vi "TestModel.vi"() -> ()   [LabVIEW 2015]
uses:
  CustomControl/Model.ctl
panel:
  in  "OK Button":bool
  in  "TestModel":T1
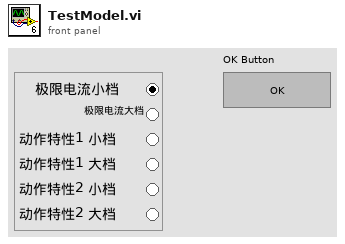
[diagram p1: front panel]
types:
  T1 = typedef "Model.ctl" = enum32{"lowLimit", "upLimit", "lowAction1", "upAction1", "lowAction2", "upAction2"}
  T2 = enum8{"Enabled", "Disabled", "Disabled and Grayed Out"}
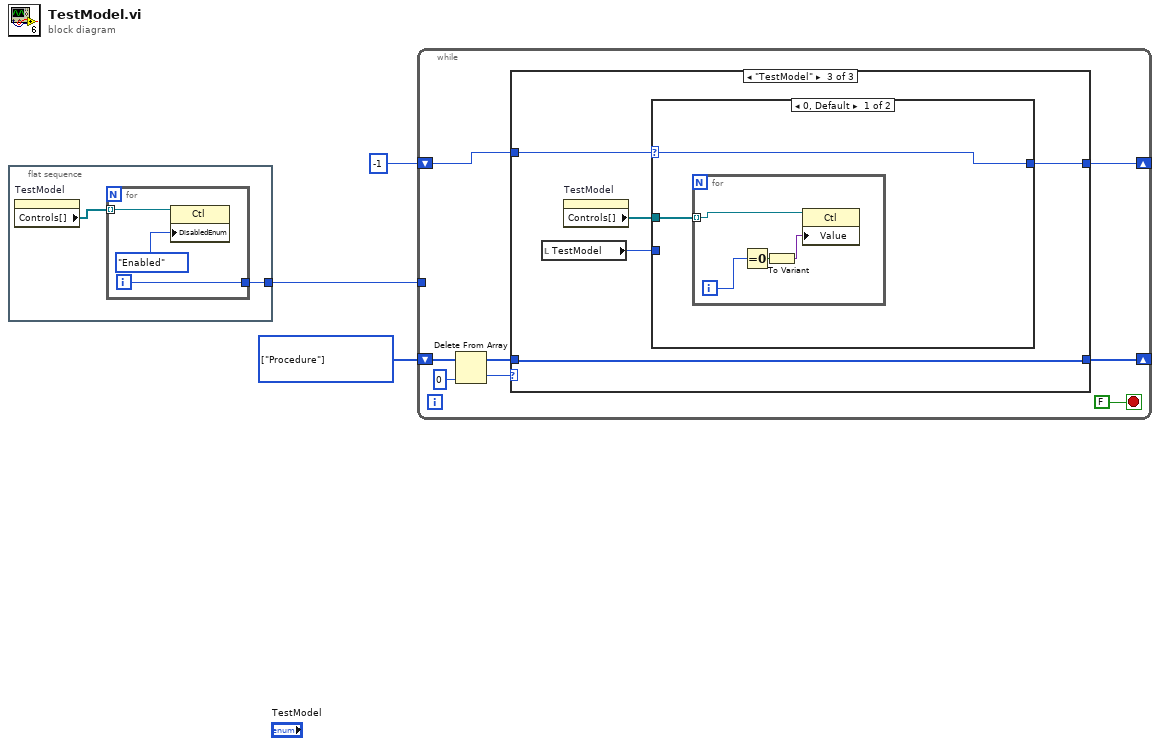
[diagram p0: block diagram]
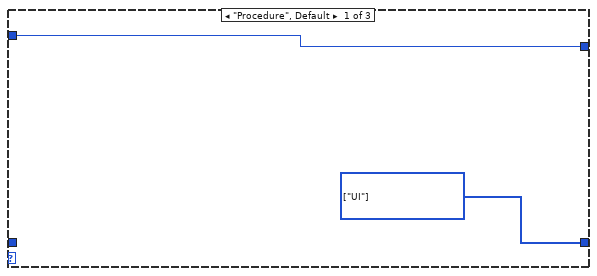
[diagram p2: hidden frame]
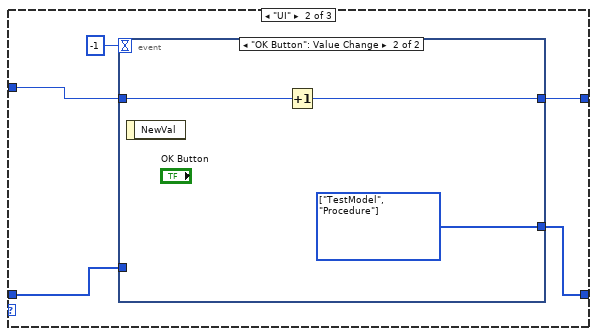
[diagram p3: hidden frame]
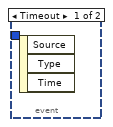
[diagram p4: hidden frame]
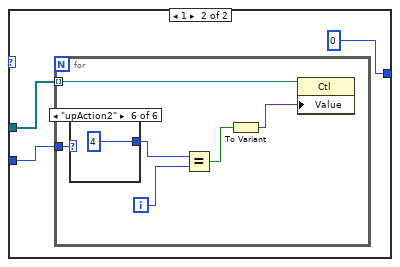
[diagram p5: hidden frame]
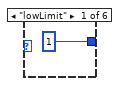
[diagram p6: hidden frame]
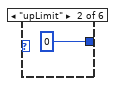
[diagram p7: hidden frame]
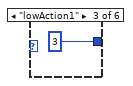
[diagram p8: hidden frame]
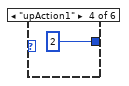
[diagram p9: hidden frame]
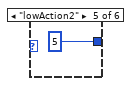
[diagram p10: hidden frame]
diagram:
  w2 = enum16{"Procedure", "UI", "TestModel"}[] [enum."Procedure"] items=["Procedure", "UI", "TestModel"]
  n1 = flat-sequence {
    tunnel: [w4] -> w1
    frame #0 {
      n2 = property on="TestModel" class="RadioBtnsControl (strict)"() -> ("Controls[]"=w5:refnum<vi>[])  [unwired: 2 in, 2 out]
      n3 = for {
        tunnel: w5 -> [w8] mode=indexing
        tunnel: [w6] -> w4
        i -> [w6]
        n4 = property class="Ctl"(reference=w8, "DisabledEnum"=T2."Enabled" ("Disabled")) -> ()  [unwired: 1 in, 2 out]
      }
    }
  }
  n5 = while {
    shift-right: [w14] -> _
    shift-left: -1 -> [w15]
    shift-right: [w10] -> _
    shift-left: w2 -> [w13]
    tunnel: w1 -> [_]
    stop <- FALSE stop-if-true
    n6 = Delete From Array(array=w13, index=0) -> (deleted portion=w12:enum16{"Procedure", "UI", "TestModel", ""}, array with subset deleted=w11:enum16{"Procedure", "UI", "TestModel", ""}[])  [unwired: 1 in]
    n7 = case shown="\"TestModel\"" w12 {
      tunnel: w15 -> [w18 w22 w28]
      tunnel: [w18 w21 w27] -> w14
      tunnel: w11 -> [_ w20 w29]
      tunnel: [w17 w19 w29] -> w10
      frame "Procedure", Default {
        w17 = enum16{"Procedure", "UI", "TestModel", ""}[] [enum."UI"] items=["Procedure", "UI", "TestModel", ""]
      }
      frame "UI" {
        n8 = event shown="[1] \"OK Button\": Value Change" {
          selector: _ -> [_ _]
          dyn-events: _ -> [_ _]
          timeout: -1 -> [_ _]
          tunnel: w22 -> [_ w26]
          tunnel: [_ w25] -> w21
          tunnel: w20 -> [_ _]
          tunnel: [_ w24] -> w19
          event Timeout {
            n9 = event-data() -> ()  [unwired: 1 in, 3 out]
          }
          event "OK Button": Value Change {
            w24 = enum16{"Procedure", "UI", "TestModel", ""}[] [enum."TestModel", enum."Procedure"] items=["Procedure", "UI", "TestModel", ""]
            n10 = event-data() -> ()  [unwired: 1 in, 1 out]
            n11 = Increment(x=w26) -> (x+1=w25:i32)
          }
        }
      }
      frame "TestModel" {
        n12 = local read "TestModel"() -> (w31:T1)
        n13 = property on="TestModel" class="RadioBtnsControl (strict)"() -> ("Controls[]"=w30:refnum<vi>[])  [unwired: 2 in, 2 out]
        n14 = case shown="0, Default" w28 {
          selector: w28 -> [w33 _]
          tunnel: w30 -> [w32 w40]
          tunnel: w31 -> [_ w39]
          tunnel: [w33 0] -> w27
          frame 0, Default {
            n15 = for {
              tunnel: w32 -> [w36] mode=indexing
              i -> [w37]
              n16 = Equal To 0?(x=w37) -> (x = 0?=w35:bool)
              n17 = To Variant(anything=w35) -> (Variant=w34:variant)
              n18 = property class="Ctl"(reference=w36, "Value"=w34) -> ()  [unwired: 1 in, 2 out]
            }
          }
          frame 1 {
            n19 = for {
              tunnel: w40 -> [w46] mode=indexing
              tunnel: w39 -> [w45]
              i -> [w43]
              n20 = case shown="\"upAction2\"" w45 {
                tunnel: [1 0 3 2 5 4] -> w44
                frame "lowLimit" {
                }
                frame "upLimit" {
                }
                frame "lowAction1" {
                }
                frame "upAction1" {
                }
                frame "lowAction2" {
                }
                frame "upAction2" {
                }
              }
              n21 = Equal?(x=w44, y=w43) -> (x = y?=w41:bool)
              n22 = To Variant(anything=w41) -> (Variant=w42:variant)
              n23 = property class="Ctl"(reference=w46, "Value"=w42) -> ()  [unwired: 1 in, 2 out]
            }
          }
        }
      }
    }
  }
